vi "PicoScope4000aExampleRapidBlockBulk.vi"() -> ()   [LabVIEW 2009]
panel:
  in  "Resolution":u16(ring) items=["12-bit", "14-bit"]
  in  "USB powered":bool
  in  "USB 3.0 on non-USB 3.0 port":bool
  in  "Trigger Settings":T1 {"Trigger Direction" items=["Rising", "Falling"]}
  in  "Serial Number":string
  in  "Use Serial Number":bool
  out "Number of Samples \nPer Capture":u32
  in  "Channel A Settings":T2 {"Range" items=["10 mV", "20 mV", "50 mV", "100 mV", "200 mV", "500 mV", "1 V", "2 V", "5 V", "10 V", "20 V", "50 V ", "100 V"]; "Coupling" items=["AC", "DC"]}
  in  "Rapid Block Acquisition Settings":T3
  out "Capture Complete":bool
  in  "Run":bool
  out "Channel A":i16[](graph)
  in  "Capture Index":i16 min=0
  in  "stop":bool
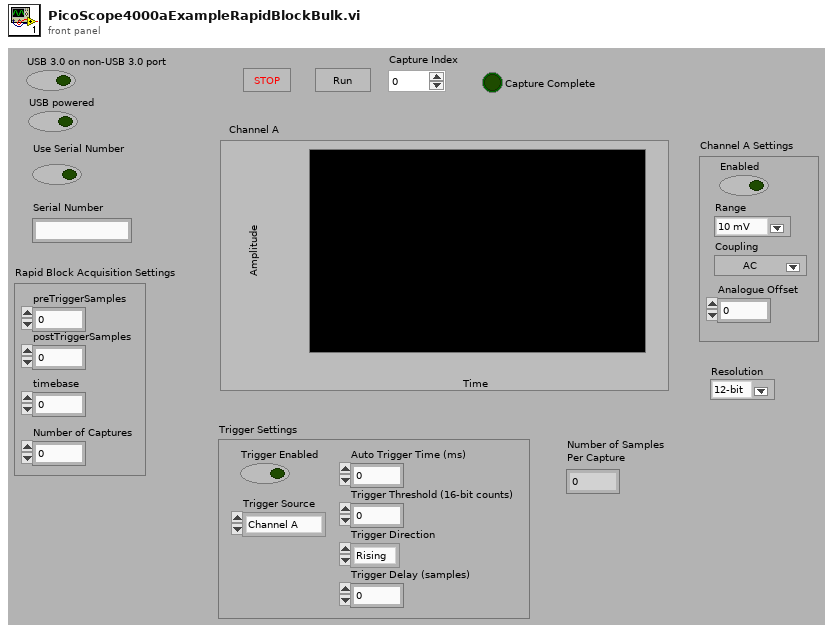
[diagram p1: front panel]
types:
  T1 = cluster{"Trigger Enabled":bool, "Trigger Source":enum16{"Channel A", "Channel B", "Channel C", "Channel D", "Channel E", "Channel F", "Channel G", "Channel H"}, "Trigger Threshold (16-bit counts)":i16, "Trigger Direction":u16, "Trigger Delay (samples)":u32, "Auto Trigger Time (ms)":i16}
  T2 = cluster{"Enabled":bool, "Coupling":i16, "Range":u16, "Analogue Offset":sgl}
  T3 = cluster{"preTriggerSamples":u32, "postTriggerSamples":u32, "timebase":u32, "Number of Captures":u32}
  T4 = cluster{"Driver Version":string, "USB Version":string, "Hardware":string, "Variant":string, "Batch and Serial":string, "Cal Date":string, "Kernel Version":string, "Digital HW Version":string, "Analogue HW Version":string, "Firmware 1":string, "Firmware 2":string, "Num. channels":i16}
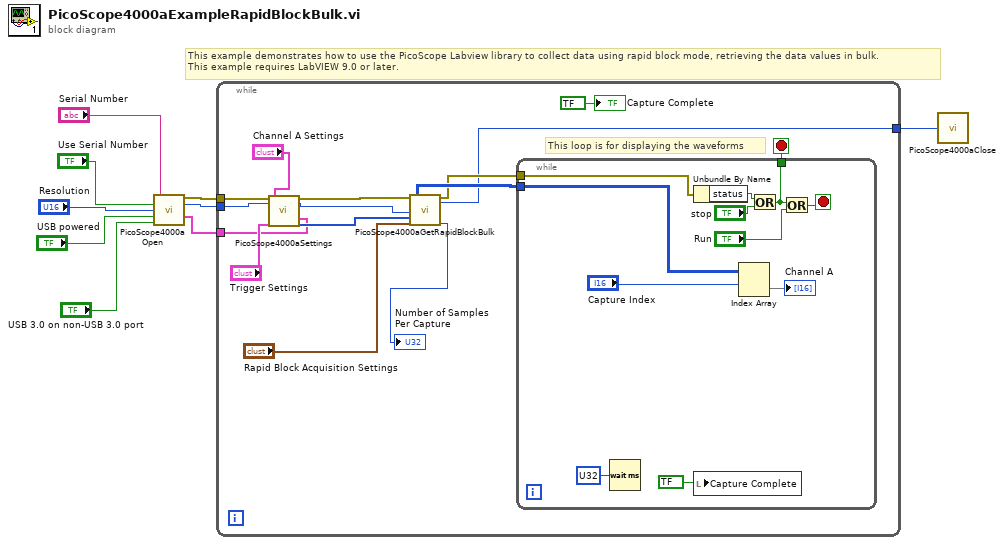
[diagram p0: block diagram]
diagram:
  # "This example demonstrates how to use the PicoScope Labview library to collect data using rapid block mode, retrieving the data values in bulk.\nThis example requires LabVIEW 9.0 or later."
  n1 = call "PicoScope4000aOpen.vi"("Serial Number"="Serial Number", "Use Serial Number"="Use Serial Number", "Resolution"="Resolution", "USB powered"="USB powered", "USB 3.0 on non-USB 3.0 port"="USB 3.0 on non-USB 3.0 port") -> ("error out"=w6:errorcluster, "handle"=w5:i16, "Unit Info"=w4:T4)  [unwired: 8 in]
  n2 = while {
    tunnel: [w17] -> w9
    tunnel: w6 -> [w22]
    tunnel: w5 -> [w20]
    tunnel: w4 -> [w10]
    stop <- w24 stop-if-true
    # "This loop is for displaying the waveforms"
    n3 = call "PicoScope4000aSettings.vi"("error in"=w22, "handle in"=w20, "Trigger Settings"="Trigger Settings", "Channel A Settings"="Channel A Settings", "Unit Info"=w10) -> ("error out"=w15:errorcluster, "handle out"=w14:i16, "Enabled array"=w12:i16[])  [unwired: 12 in]
    n4 = call "PicoScope4000aGetRapidBlockBulk.vi"("error in"=w15, "handle in"=w14, "Enabled array"=w12, "Rapid Block Acquisition Settings"="Rapid Block Acquisition Settings") -> ("Channel A Buffer"=w19:i16[][], "error out"=w18:errorcluster, "handle out"=w17:i16, "Num samples"=→"Number of Samples \nPer Capture":u32)  [unwired: 5 in, 7 out]
    n5 = while {
      tunnel: [w34] -> w24
      tunnel: w19 -> [w27]
      tunnel: w18 -> [w29]
      stop <- w33 stop-if-true
      n6 = Wait (ms)(milliseconds to wait=u32 ?) -> ()  [unwired: 1 out]
      n7 = Unbundle By Name(w29) -> ("status"=w28:bool)
      n8 = local write "Capture Complete"(bool ? ("Capture Complete")) -> ()
      n9 = Index Array(array=w27, index (row)="Capture Index") -> (element=→"Channel A":i16[])  [unwired: 1 in]
      n10 = Or(x=w28, y="stop") -> (x .or. y?=w34:bool)
      n11 = Or(x=w34, y="Run") -> (x .or. y?=w33:bool)
    }
    "Capture Complete" <- bool ? ("Capture Complete")
  }
  n12 = call "PicoScope4000aClose.vi"("handle"=w9) -> ()
